vi "PH_Tektronix_7000.Evt Call get Channel Configuration.vi"(0 "i ref in":refnum<vi>, 1 "Instance":string="N/A", 2 "Channel":u16(ring) items=["Channel 1", "Channel 2", "Channel 3", "Channel 4", "Math 1", "Math 2", "Math 3", "Math 4", "Reference 1", "Reference 2", "Reference 3", "Reference 4"], 5 "error in (no error)":errorcluster) -> (14 "i ref out":refnum<vi>, 19 "error out":errorcluster)   [LabVIEW 2014, in "PH_Tektronix_7000.lvlib"]
doc: "This VI calls sets a simple call."
uses:
  PH_Tektronix_7000.lvlib
  CSCore/CSSystem/CoreLib/CoreLib.short 2 byte array.vi
  CSCore/CSSystem/CoreLib/CoreLib.lvlib
  CSCore/BaseProcess/BaseProcess.lvlib
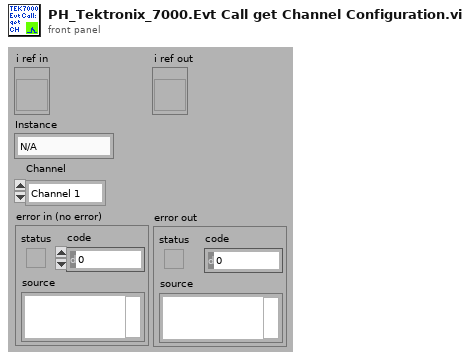
[diagram p1: front panel]
types:
  T1 = typedef "CoreDefs.rawDataType.ctl" = i8[]
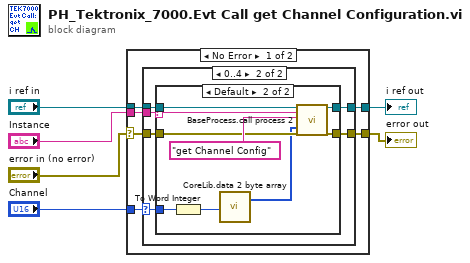
[diagram p0: block diagram]
diagram:
  n1 = case shown="No Error" "error in (no error)" {
    selector: "error in (no error)" -> [w8 w32]
    tunnel: [w12 w33] -> w6
    tunnel: [w11 w32] -> w5
    tunnel: "i ref in" -> [w10 w33]
    tunnel: "Channel" -> [w7 _]
    tunnel: "Instance" -> [w9 _]
    frame No Error {
      n2 = case shown="0..4" w7 {
        selector: w7 -> [_ w15]
        tunnel: [w14 w20] -> w12
        tunnel: [w13 w19] -> w11
        tunnel: w10 -> [w14 w18]
        tunnel: w9 -> [_ w17]
        tunnel: w8 -> [w13 w16]
        frame Default {
        }
        frame 0..4 {
          n3 = case shown="Default" w17 {
            selector: w17 -> [_ w26]
            tunnel: [w21 w30] -> w20
            tunnel: [w22 w29] -> w19
            tunnel: w18 -> [w21 w28]
            tunnel: w16 -> [w22 w27]
            tunnel: w15 -> [_ w25]
            frame "N/A" {
            }
            frame Default {
              n4 = To Word Integer(number=w25) -> (16bit integer=w24:i16)
              n5 = call-poly "CoreLib.data 2 byte array.vi"("i16"=w24) -> ("byteArray out"=w23:T1)  [unwired: 18 in]
              n6 = call "BaseProcess.call process 2.vi"("i ref in"=w28, "Object"=w26, "Selector"="get Channel Config", "Data"=w23, "error in (no error)"=w27) -> ("i ref out"=w30:refnum<vi>, "error out"=w29:errorcluster)  [unwired: 13 in]
            }
          }
        }
      }
    }
    frame Error {
    }
  }
  "i ref out" <- w6
  "error out" <- w5
